vi "Create Unique Channel Names.vi"(8 "error in":errorcluster, 11 "SwitchMatrix in":refnum<class "SwitchMatrix.lvclass">) -> (0 "error out":errorcluster, 3 "SwitchMatrix out":refnum<class "SwitchMatrix.lvclass">)   [LabVIEW 2019, in "SwitchMatrix.lvlib" / "SwitchMatrix.lvclass"]
uses:
  Library/SwitchMatrix.lvclass
  C:/Users/Public/Documents/Development/builds/Engine/Monitored Actor.lvlibp/Monitored Actor/Monitored Actor/Monitored Actor.lvclass
  Library/SwitchMatrix.lvclass/SwitchMatrix.ctl
  builds/Engine/Monitored Actor.lvlibp/Monitored Actor/Monitored Actor/Read Actor Label.vi
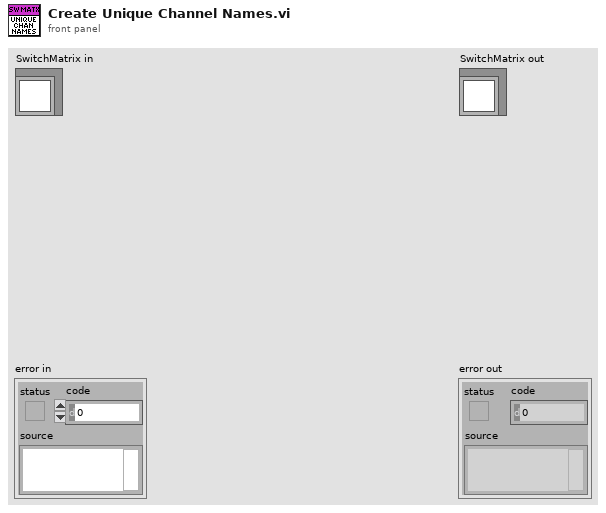
[diagram p1: front panel]
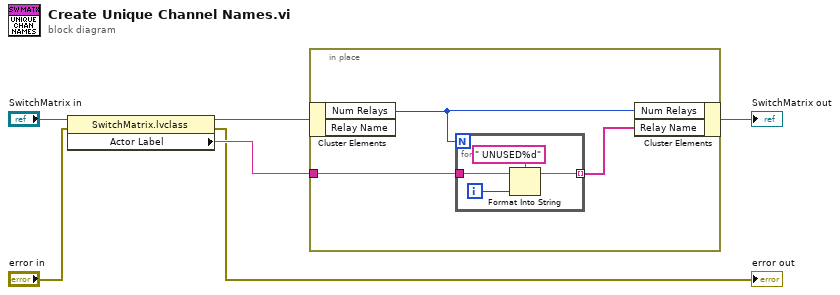
[diagram p0: block diagram]
diagram:
  n1 = property class="SwitchMatrix.lvclass"(reference="SwitchMatrix in", error in="error in") -> (reference out=w3:refnum<class "SwitchMatrix.lvclass">, error out=→"error out":errorcluster, "Actor Label"=w4:string)
  n2 = in-place {
    in-place-border: w4 -> [w8]
    n3 = in-place-cluster #1(w3) -> ("Num Relays"=w7:i32)  [unwired: 1 out]
    n4 = for {
      N: w7 -> [_]
      tunnel: w8 -> [w13]
      tunnel: [w10] -> w9 mode=indexing
      i -> [w11]
      n5 = Format Into String(format string=" UNUSED%d", initial string=w13, w11) -> (resulting string=w10:string)  [unwired: 1 in, 1 out]
    }
    n6 = in-place-cluster #1("Num Relays"=w7, "Relay Name"=w9) -> (→"SwitchMatrix out":refnum<class "SwitchMatrix.lvclass">)
  }
